vi "Load Image (Core).vi"(8 "error in (no error)":errorcluster, 11 "Path In":string) -> (0 "error out":errorcluster, 2 "Picture":T1, 3 "Path Out":string)   [LabVIEW 2020, in "G-Image.lvlib"]
doc: "Retrieve audio file information. Some codecs (mp3) require the entire file be parsed to accurately determine the length, which can take time for very large files.\n\nSupported codecs: flac, mp3, ogg (vorbis), and wav."
uses:
  G-Image.lvlib
  <vilib>/picture/picture.llb/imagedata.ctl
  <vilib>/Utility/file.llb/Application Directory.vi
  <vilib>/Utility/error.llb/Error Cluster From Error Code.vi
  lib/g_image_32.dll
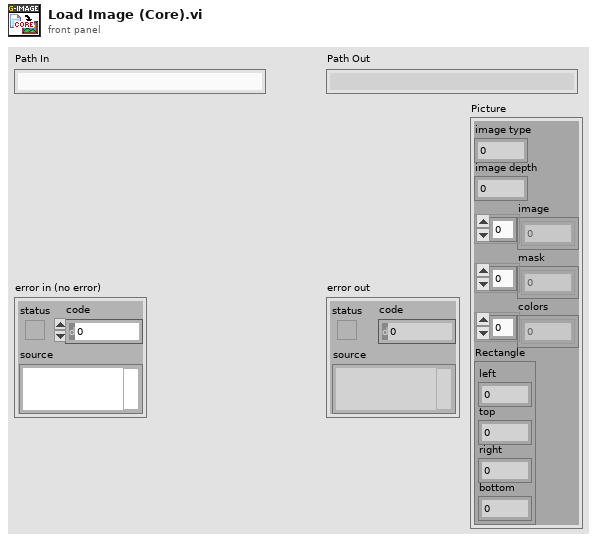
[diagram p1: front panel]
types:
  T1 = typedef "imagedata.ctl" = cluster{"image type":i32, "image depth":i32, "image":u8[], "mask":u8[], "colors":u32[], "Rectangle":cluster{"left":i16, "top":i16, "right":i16, "bottom":i16}}
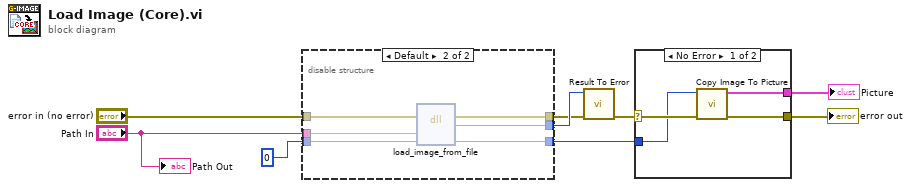
[diagram p0: block diagram]
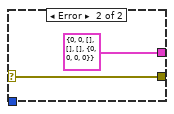
[diagram p2: hidden frame]
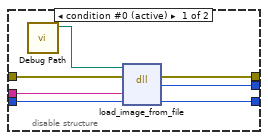
[diagram p3: hidden frame]
diagram:
  n1 = disable-structure shown="Default" {
    disable-tunnel: [w15 w22] -> w6
    disable-tunnel: "error in (no error)" -> [w14 w21]
    disable-tunnel: "Path In" -> [w13 w20]
    disable-tunnel: [w12 w19] -> w7
    disable-tunnel: [w11 w17] -> w2
    disable-tunnel: i64 0 ("count") -> [w10 w18]
    frame condition #0 (active) {
      n2 = call "Debug Path.vi"() -> ("Debug Path"=w16:path)  [unwired: 11 in]
      n3 = dll-call lib="?" fn="load_image_from_file"(path in=w16, error in=w14, "file_name"=w13, "image_out"=w10) -> (error out=w15:errorcluster, "result"=w12:i32, "image_out"=w11:i64)  [unwired: 2 in, 1 out]
    }
    frame condition #1 {
      n4 = dll-call lib="C:/github/dataflowg/g-image/src/LabVIEW/G-Image/lib/g_image_*.*" fn="load_image_from_file"(error in=w21, "file_name"=w20, "image_out"=w18) -> (error out=w22:errorcluster, "result"=w19:i32, "image_out"=w17:i64)  [unwired: 3 in, 1 out]
    }
  }
  n5 = call "Result To Error.vi"("error in (no error)"=w6, "Result Code"=w7) -> ("error out"=w5:errorcluster)  [unwired: 9 in]
  n6 = case shown="No Error" w5 {
    selector: w5 -> [w26 w28]
    tunnel: [w24 w28] -> w9
    tunnel: w2 -> [w25 _]
    tunnel: [w23 T1 {"image type"=0, "image depth"=0, "image"=[], "mask"=[], "colors"=[], "Rectangle"={"left"=0, "top"=0, "right"=0, "bottom"=0}} ("Image")] -> w1
    frame No Error {
      n7 = call "Copy Image To Picture.vi"("error in (no error)"=w26, "image_ptr"=w25) -> ("error out"=w24:errorcluster, "Picture"=w23:T1)  [unwired: 8 in]
    }
    frame Error {
    }
  }
  "error out" <- w9
  "Picture" <- w1
  "Path Out" <- "Path In"
